vi "m_file_V2021.vi"() -> ()   [LabVIEW 2021]
panel:
  out "Diff":dbl
  out "Sum":dbl
  in  "X2":dbl=10.0
  in  "X1":dbl=50.0
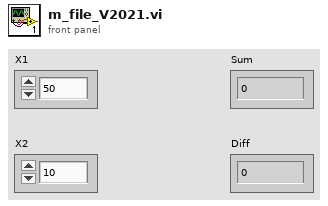
[diagram p1: front panel]
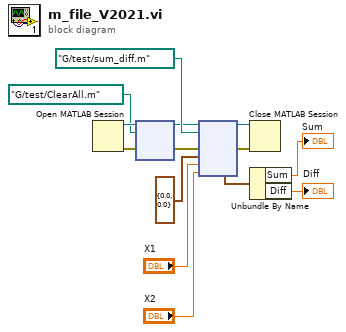
[diagram p0: block diagram]
diagram:
  n1 = Open MATLAB Session() -> (8:w5:refnum<k37>, 11:w4:errorcluster)  [unwired: 2 in]
  n2 = node(w5, path "G:/test/ClearAll.m" ("source file path"), w4) -> (w3:refnum<k37>, w2:errorcluster)  [unwired: 3 in, 2 out]
  n3 = node(w3, path "G:/test/sum_diff.m" ("source file path"), w2, cluster{"Sum":dbl, "Diff":dbl} {"Sum"=0.0, "Diff"=0.0} ("Cluster"), "X1", "X2") -> (w14:refnum<k37>, w13:errorcluster, w9:cluster{"Sum":dbl, "Diff":dbl})  [unwired: 3 in, 2 out]
  n4 = Close MATLAB Session(0:w14, 3:w13) -> ()  [unwired: 1 out]
  n5 = Unbundle By Name(w9) -> ("Sum"=→"Sum":dbl, "Diff"=→"Diff":dbl)
